vi "gates all channels.vi"() -> ()   [LabVIEW 2018]
uses:
  <userlib>/_OpenG.lib/array/array.llb/Filter 1D Array with Scalar (String)__ogtk.vi
  <vilib>/Utility/file.llb/Write Delimited Spreadsheet (string).vi
panel:
  out "Array 2":tag[][](array[tag])
  out "error out":errorcluster
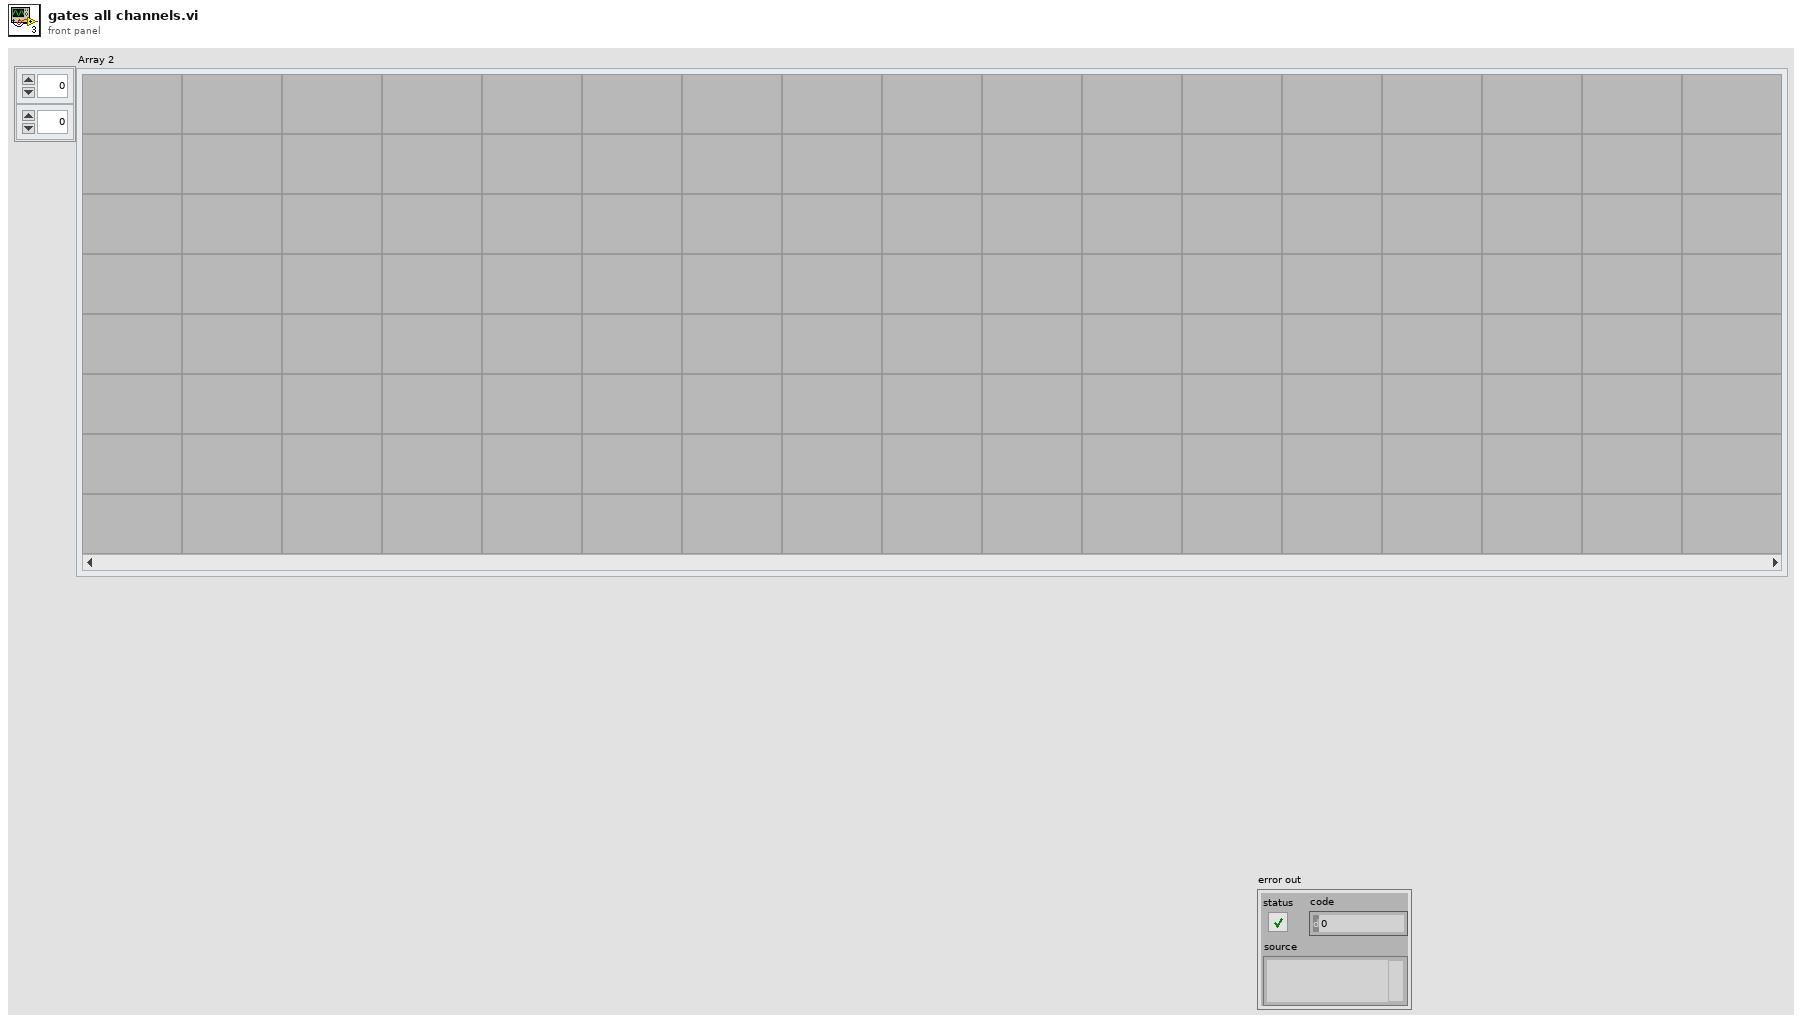
[diagram p1: front panel]
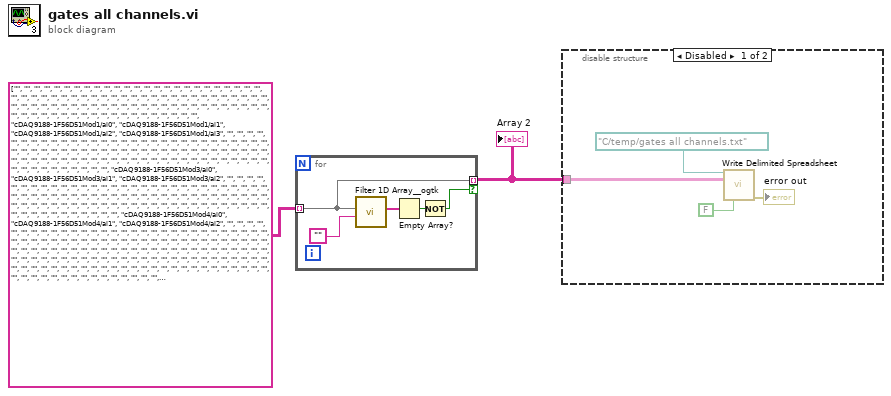
[diagram p0: block diagram]
diagram:
  n1 = for {
    tunnel: tag[][] [["", "", "", "", "", "", "", "", "", "", "", "", "", "", "", ""], ["", "", "", "", "", "", "", "", "", "", "", "", "", "", "", ""], ["", "", "", "", "", "", "", "", "", "", "", "", "", "", "", ""], ["", "", "", "", "", "", "", "", "", "", "", "", "", "", "", ""], ["", "", "", "", "", "", "", "", "", "", "", "", "", "", "", ""], ["", "", "", "", "", "", "", "", "", "", "", "", "", "", "", ""], ["cDAQ9188-1F56D51Mod1/ai0", "cDAQ9188-1F56D51Mod1/ai1", "cDAQ9188-1F56D51Mod1/ai2", "cDAQ9188-1F56D51Mod1/ai3", "", "", "", "", "", "", "", "", "", "", "", ""], ["", "", "", "", "", "", "", "", "", "", "", "", "", "", "", ""], ["", "", "", "", "", "", "", "", "", "", "", "", "", "", "", ""], ["", "", "", "", "", "", "", "", "", "", "", "", "", "", "", ""], ["", "", "", "", "", "", "", "", "", "", "", "", "", "", "", ""], ["", "", "", "", "", "", "", "", "", "", "", "", "", "", "", ""], ["cDAQ9188-1F56D51Mod3/ai0", "cDAQ9188-1F56D51Mod3/ai1", "cDAQ9188-1F56D51Mod3/ai2", "", "", "", "", "", "", "", "", "", "", "", "", ""], ["", "", "", "", "", "", "", "", "", "", "", "", "", "", "", ""], ["", "", "", "", "", "", "", "", "", "", "", "", "", "", "", ""], ["", "", "", "", "", "", "", "", "", "", "", "", "", "", "", ""], ["", "", "", "", "", "", "", "", "", "", "", "", "", "", "", ""], ["", "", "", "", "", "", "", "", "", "", "", "", "", "", "", ""], ["cDAQ9188-1F56D51Mod4/ai0", "cDAQ9188-1F56D51Mod4/ai1", "cDAQ9188-1F56D51Mod4/ai2", "", "", "", "", "", "", "", "", "", "", "", "", ""], ["", "", "", "", "", "", "", "", "", "", "", "", "", "", "", ""], ["", "", "", "", "", "", "", "", "", "", "", "", "", "", "", ""], ["", "", "", "", "", "", "", "", "", "", "", "", "", "", "", ""], ["", "", "", "", "", "", "", "", "", "", "", "", "", "", "", ""], ["", "", "", "", "", "", "", "", "", "", "", "", "", "", "", ""], ["", "", "", "", "", "", "", "", "", "", "", "", "", "", "", ""], ["", "", "", "", "", "", "", "", "", "", "", "", "", "", "", ""], ["", "", "", "", "", "", "", "", "", "", "", "", "", "", "", ""], ["", "", "", "", "", "", "", "", "", "", "", "", "", "", "", ""], ["cDAQ9188-1F56D51Mod6/ctr0", "cDAQ9188-1F56D51Mod6/ctr1", "cDAQ9188-1F56D51Mod6/ctr2", "cDAQ9188-1F56D51Mod6/ctr3", "cDAQ9188-1F56D51Mod6/ctr4", "cDAQ9188-1F56D51Mod6/ctr5", "cDAQ9188-1F56D51Mod6/ctr6", "cDAQ9188-1F56D51Mod6/ctr7", "", "", "", "", "", "", "", ""], ["", "", "", "", "", "", "", "", "", "", "", "", "", "", "", ""], ["", "", "", "", "", "", "", "", "", "", "", "", "", "", "", ""], ["cDAQ9188-1F56D51Mod7/ao0", "cDAQ9188-1F56D51Mod7/ao1", "cDAQ9188-1F56D51Mod7/ao2", "cDAQ9188-1F56D51Mod7/ao3", "", "", "", "", "", "", "", "", "", "", "", ""], ["", "", "", "", "", "", "", "", "", "", "", "", "", "", "", ""], ["", "", "", "", "", "", "", "", "", "", "", "", "", "", "", ""], ["", "", "", "", "", "", "", "", "", "", "", "", "", "", "", ""], ["", "", "", "", "", "", "", "", "", "", "", "", "", "", "", ""], ["", "", "", "", "", "", "", "", "", "", "", "", "", "", "", ""], ["", "", "", "", "", "", "", "", "", "", "", "", "", "", "", ""], ["cDAQ9188-1F56D51Mod8/port0/line0", "cDAQ9188-1F56D51Mod8/port0/line1", "cDAQ9188-1F56D51Mod8/port0/line2", "cDAQ9188-1F56D51Mod8/port0/line3", "cDAQ9188-1F56D51Mod8/port0/line4", "cDAQ9188-1F56D51Mod8/port0/line5", "cDAQ9188-1F56D51Mod8/port0/line6", "cDAQ9188-1F56D51Mod8/port0/line7", "cDAQ9188-1F56D51Mod8/port0/line8", "cDAQ9188-1F56D51Mod8/port0/line9", "cDAQ9188-1F56D51Mod8/port0/line10", "cDAQ9188-1F56D51Mod8/port0/line11", "cDAQ9188-1F56D51Mod8/port0/line12", "cDAQ9188-1F56D51Mod8/port0/line13", "cDAQ9188-1F56D51Mod8/port0/line14", "cDAQ9188-1F56D51Mod8/port0/line15"], ["cDAQ9188-1F56D51Mod8/port1/line0", "cDAQ9188-1F56D51Mod8/port1/line1", "cDAQ9188-1F56D51Mod8/port1/line2", "cDAQ9188-1F56D51Mod8/port1/line3", "cDAQ9188-1F56D51Mod8/port1/line4", "cDAQ9188-1F56D51Mod8/port1/line5", "cDAQ9188-1F56D51Mod8/port1/line6", "cDAQ9188-1F56D51Mod8/port1/line7", "cDAQ9188-1F56D51Mod8/port1/line8", "cDAQ9188-1F56D51Mod8/port1/line9", "cDAQ9188-1F56D51Mod8/port1/line10", "cDAQ9188-1F56D51Mod8/port1/line11", "cDAQ9188-1F56D51Mod8/port1/line12", "cDAQ9188-1F56D51Mod8/port1/line13", "cDAQ9188-1F56D51Mod8/port1/line14", "cDAQ9188-1F56D51Mod8/port1/line15"], ["", "", "", "", "", "", "", "", "", "", "", "", "", "", "", ""], ["", "", "", "", "", "", "", "", "", "", "", "", "", "", "", ""]] ("Array 2") -> [w5] mode=indexing
    tunnel: [w5] -> w1 mode=indexing if=w3
    n2 = call-poly <userlib>:"Filter 1D Array__ogtk.vi"("items to filter"="", "array"=w5) -> ("filtered array"=w6:string[])  [unwired: 4 in, 1 out]
    n3 = Empty Array?(array=w6) -> (empty?=w4:bool)
    n4 = Not(x=w4) -> (.not. x?=w3:bool)
  }
  "Array 2" <- w1
  n5 = disable-structure shown="Disabled" {
    disable-tunnel: w1 -> [w8 _]
    frame Disabled {
      n6 = call-poly <vilib>:"Write Delimited Spreadsheet.vi"("file path (dialog if empty)"=path "C:/temp/gates all channels.txt", "2D data"=w8, "transpose? (no:F)"=FALSE) -> ("error out"=→"error out":errorcluster)  [unwired: 11 in, 1 out]
    }
    frame Enabled {
    }
  }
